vi "Set NISync Plugin Timekeeper.vi"(8 "error in (no error)":errorcluster, 11 "RT Data Cluster in":T1={"Timekeeper hdl"="", "clkDisc session"=variant, "Compiled Data"={"SyncMod?"=FALSE, "SyncMod"="", "ConnectionSettings"={"Mode"=enum."Generate sample clock", "pxitrig"=FALSE, "pfi0"=FALSE, "pfi1"=FALSE, "pfi2"=FALSE, "External Pin"=enum."PFI0", "Routes"=[]}, "TimeKeeper"="", "ScanOffset(%)"=0.0, "StartDelay(s)"=0, "Time Ref Settings"={"Time Reference"=enum."GPS", "Priority 1"=0, "Priority 2"=0, "IRIG type"=enum."IRIGB AM", "Terminal"="", "PPSSetTime"=FALSE, "Start Time"=timestamp(0 s since 1904-01-01)}, "FIFO Locations"={"SysTime"=[], "TimeRef"=[], "Status"=[]}}, "OutputsData"=[], "OutputsFIFO"=refnum, "Scan Period"=0, "Timekeeper type"=enum."6683", "SyncMod type"=enum."6683", "SyncMod hdl"=""} {"Compiled Data"."Time Ref Settings"."Priority 2" min=0 max=255; "Compiled Data"."Time Ref Settings"."Priority 1" min=0 max=255}) -> (0 "error out":errorcluster, 3 "RT Data Cluster out":T1={"Timekeeper hdl"="", "clkDisc session"=variant, "Compiled Data"={"SyncMod?"=FALSE, "SyncMod"="", "ConnectionSettings"={"Mode"=enum."Generate sample clock", "pxitrig"=FALSE, "pfi0"=FALSE, "pfi1"=FALSE, "pfi2"=FALSE, "External Pin"=enum."PFI0", "Routes"=[]}, "TimeKeeper"="", "ScanOffset(%)"=0.0, "StartDelay(s)"=0, "Time Ref Settings"={"Time Reference"=enum."GPS", "Priority 1"=0, "Priority 2"=0, "IRIG type"=enum."IRIGB AM", "Terminal"="", "PPSSetTime"=FALSE, "Start Time"=timestamp(0 s since 1904-01-01)}, "FIFO Locations"={"SysTime"=[], "TimeRef"=[], "Status"=[]}}, "OutputsData"=[], "OutputsFIFO"=refnum, "Scan Period"=0, "Timekeeper type"=enum."6683", "SyncMod type"=enum."6683", "SyncMod hdl"=""} {"Compiled Data"."Time Ref Settings"."Priority 2" min=0 max=255; "Compiled Data"."Time Ref Settings"."Priority 1" min=0 max=255})   [LabVIEW 2018, in "Chassis TimeSync Engine.lvlib"]
uses:
  Chassis TimeSync Engine.lvlib
  RT Data Cluster.ctl
  mdevClkDisc.llb/_clkDisc_session.ctl
  Shared/Compiled Data.ctl
  Shared/Connection Settings.ctl
  Shared/Mode.ctl
  Shared/External Pin.ctl
  Shared/Routes.ctl
  Shared/Route.ctl
  Shared/Time Ref Settings.ctl
  Shared/Time Reference.ctl
  Shared/IRIG Type.ctl
  timekeeper type.ctl
  <vilib>/Utility/config.llb/NI_LVConfig.lvlib
  <vilib>/Utility/config.llb/Read Key (String).vi
  <vilib>/Utility/config.llb/Write Key (String).vi
  Shared/Chassis TimeSync Shared.lvlib
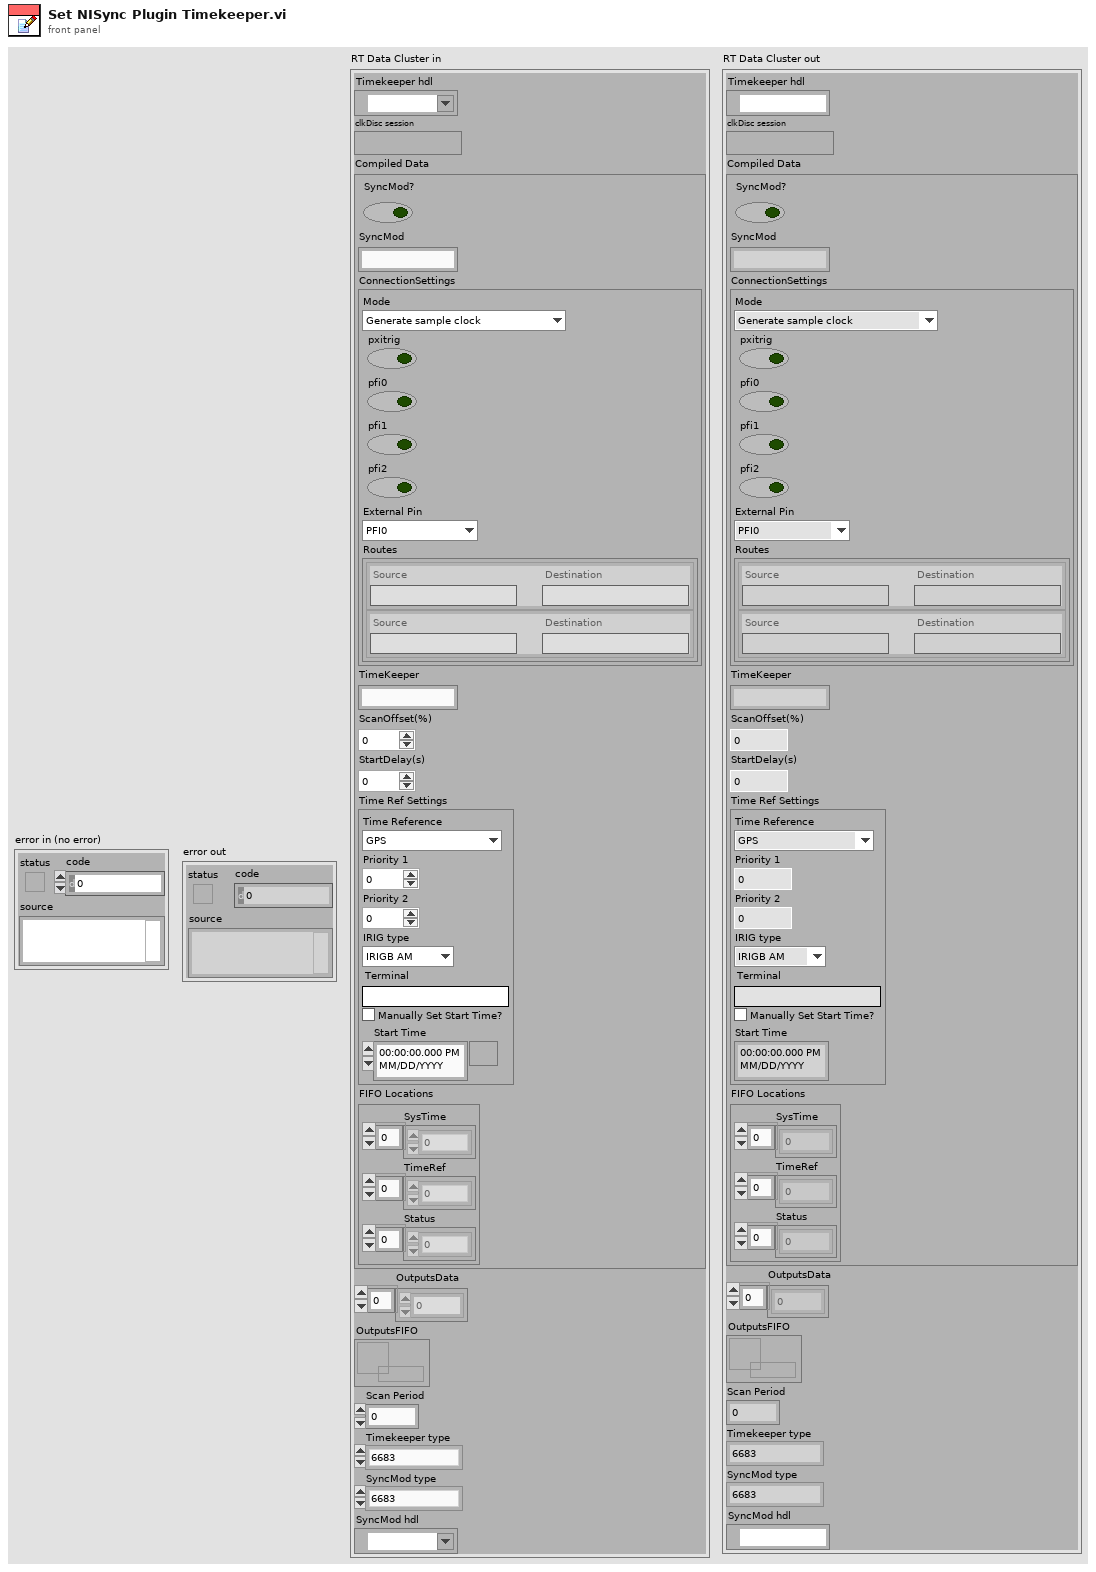
[diagram p1: front panel]
types:
  T1 = typedef "Chassis TimeSync Engine.lvlib/RT Data Cluster.ctl" = cluster{"Timekeeper hdl":refnum<k15>, "clkDisc session":T2, "Compiled Data":T3, "OutputsData":dbl[], "OutputsFIFO":refnum<k33>, "Scan Period":u32, "Timekeeper type":T12, "SyncMod type":T12, "SyncMod hdl":refnum<k15>}
  T2 = typedef "_clkDisc_session.ctl" = variant
  T3 = typedef "Chassis TimeSync Shared.lvlib/Compiled Data.ctl" = cluster{"SyncMod?":bool, "SyncMod":string, "ConnectionSettings":T4, "TimeKeeper":string, "ScanOffset(%)":dbl, "StartDelay(s)":u16, "Time Ref Settings":T9, "FIFO Locations":cluster{"SysTime":i32[], "TimeRef":i32[], "Status":i32[]}}
  T4 = typedef "Chassis TimeSync Shared.lvlib/Connection Settings.ctl" = cluster{"Mode":T5, "pxitrig":bool, "pfi0":bool, "pfi1":bool, "pfi2":bool, "External Pin":T6, "Routes":T7}
  T5 = typedef "Chassis TimeSync Shared.lvlib/Mode.ctl" = enum16{"Generate sample clock", "Route sample clock out of chassis", "Route sample clock into chassis", "Custom routes"}
  T6 = typedef "Chassis TimeSync Shared.lvlib/External Pin.ctl" = enum16{"PFI0", "PFI1", "PFI2"}
  T7 = typedef "Chassis TimeSync Shared.lvlib/Routes.ctl" = T8[]
  T8 = typedef "Chassis TimeSync Shared.lvlib/Route.ctl" = cluster{"Source":string, "Destination":string}
  T9 = typedef "Chassis TimeSync Shared.lvlib/Time Ref Settings.ctl" = cluster{"Time Reference":T10, "Priority 1":i32, "Priority 2":i32, "IRIG type":T11, "Terminal":string, "PPSSetTime":bool, "Start Time":timestamp}
  T10 = typedef "Chassis TimeSync Shared.lvlib/Time Reference.ctl" = enum16{"GPS", "IRIG", "PPS", "1588 Ordinary Clock", "PXI Chassis Clock", "Free Running (Internal)"}
  T11 = typedef "Chassis TimeSync Shared.lvlib/IRIG Type.ctl" = enum16{"IRIGB DC", "IRIGB AM"}
  T12 = typedef "Chassis TimeSync Engine.lvlib/timekeeper type.ctl" = enum16{"6683", "6683H", "6682", "6682H", "non-timekeeper", "timekeeper"}
  T13 = typedef "NI_LVConfig.lvlib/Config Data RefNum.ctl" = refnum<k1>
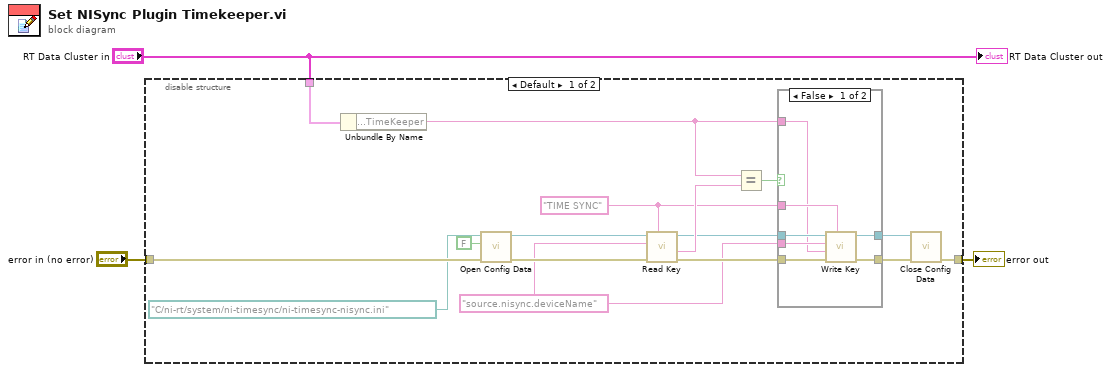
[diagram p0: block diagram]
diagram:
  n1 = disable-structure shown="Default" {
    disable-tunnel: "error in (no error)" -> [w19 w29]
    disable-tunnel: "RT Data Cluster in" -> [w12 _]
    disable-tunnel: [w4 w29] -> w1
    frame condition #0 {
      w8 = "source.nisync.deviceName" ("section")
      w9 = "TIME SYNC" ("section")
      n2 = Unbundle By Name(w12) -> ("Compiled Data.TimeKeeper"=w7:string)
      n3 = call <vilib>:"Open Config Data.vi"("error in (no error)"=w19, "create file if necessary (T)"=FALSE, "configuration file path"=path "C:/ni-rt/system/ni-timesync/ni-timesync-nisync.ini") -> ("error out"=w16:errorcluster, "refnum"=w15:T13)  [unwired: 6 in, 1 out]
      n4 = call-poly <vilib>:"Read Key.vi"("section"=w9, "error in (no error)"=w16, "key"=w8, "refnum"=w15) -> ("error out"=w14:errorcluster, "value"=w13:string, "refnum out"=w10:T13)  [unwired: 4 in, 1 out]
      n5 = Equal?(x=w7, y=w13) -> (x = y?=w11:bool)
      n6 = case shown="False" w11 {
        tunnel: w14 -> [w26 w27]
        tunnel: w10 -> [w25 w28]
        tunnel: w9 -> [w24 _]
        tunnel: w8 -> [w23 _]
        tunnel: w7 -> [w22 _]
        tunnel: [w21 w27] -> w6
        tunnel: [w20 w28] -> w5
        frame False {
          n7 = call-poly <vilib>:"Write Key.vi"("section"=w24, "error in (no error)"=w26, "value"=w22, "key"=w23, "refnum"=w25) -> ("error out"=w21:errorcluster, "refnum out"=w20:T13)  [unwired: 4 in, 1 out]
        }
        frame True {
        }
      }
      n8 = call <vilib>:"Close Config Data.vi"("error in (no error)"=w6, "refnum"=w5) -> ("error out"=w4:errorcluster)  [unwired: 8 in, 1 out]
    }
    frame condition #1 (active) {
    }
  }
  "error out" <- w1
  "RT Data Cluster out" <- "RT Data Cluster in"
